vi "Calculate MF.vi"(8 "error in (no error)":errorcluster, 11 "MeritFactor in":refnum<class "MeritFactor.lvclass">) -> (0 "error out":errorcluster, 3 "MeritFactor out":refnum<class "MeritFactor.lvclass">)   [LabVIEW 2012, in "MeritFactor.lvclass"]
uses:
  MeritFactor.lvclass
  MeritFactor.lvclass/MeritFactor.ctl
  <vilib>/Analysis/baseanly.llb/Mean (DBL).vi
  <vilib>/vision/NI_Vision_Development_Module.lvlib
  <vilib>/Analysis/NI_AALBase.lvlib
panel:
  in  "Keep/Replace Value (Replace)":bool
  out "System Waveform Graph 2":T1(graph)
  out "time lapse":dbl
  out "System Waveform Graph":u32[](graph)
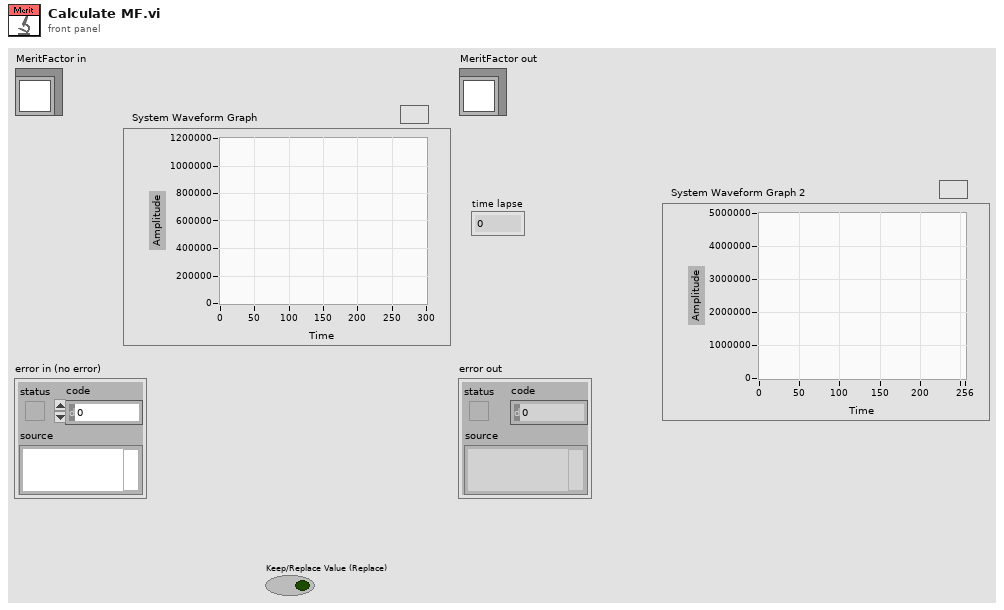
[diagram p1: front panel]
types:
  T1 = cluster{"Starting Value":sgl, "Incremental Value":sgl, "Histogram":u32[]}
  T2 = typedef "MeritFactor.lvclass/merit factor type.ctl" = enum16{"Full frame intensity", "Brightest pixels intensity", "Contrast (Keller & Stelzer)", "Contrast", "Above-threshold average"}
  T3 = typedef "IMAQ Image.ctl" = refnum<image>
  T4 = cluster{"histogram":u32[], "Minimal Value":sgl, "Maximal Value":sgl, "Starting Value":sgl, "Interval Width":sgl, "Mean Value":sgl, "Standard  Variation":sgl, "Area (pixels)":i32}
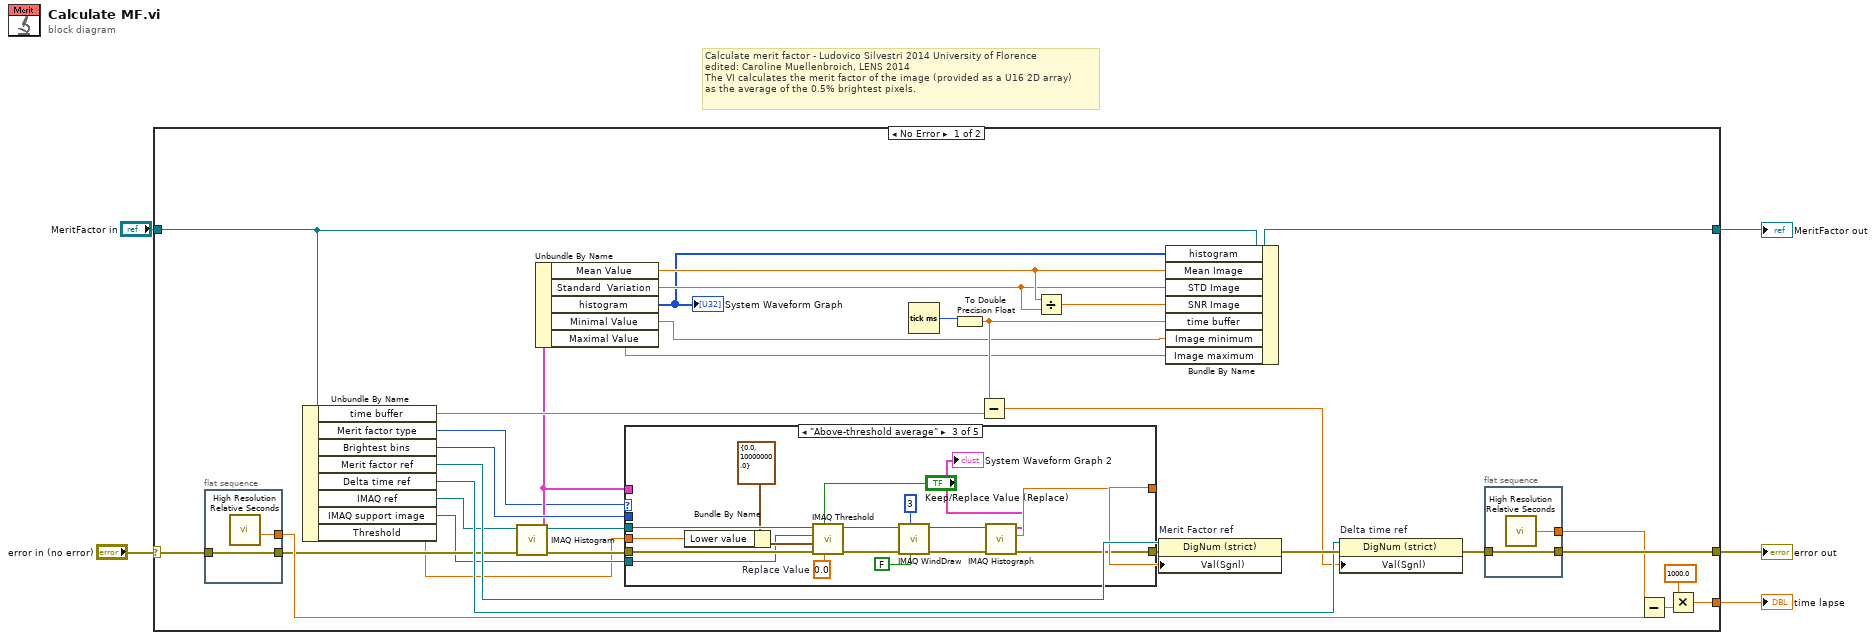
[diagram p0: block diagram]
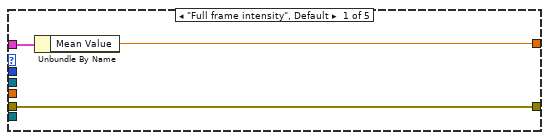
[diagram p2: hidden frame]
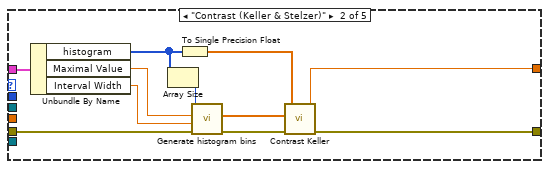
[diagram p3: hidden frame]
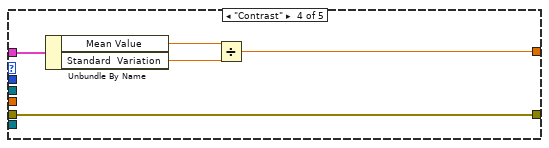
[diagram p4: hidden frame]
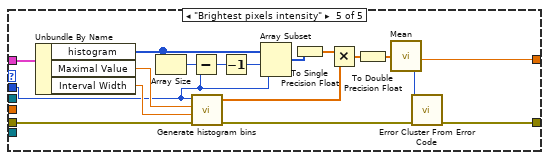
[diagram p5: hidden frame]
diagram:
  # "Calculate merit factor - Ludovico Silvestri 2014 University of Florence\nedited: Caroline Muellenbroich, LENS 2014\nThe VI calculates the merit factor of the image (provided as a U16 2D array)\nas the average of the 0.5% brightest pixels."
  n1 = case shown="No Error" "error in (no error)" {
    selector: "error in (no error)" -> [w32 w98]
    tunnel: [w30 w98] -> w4
    tunnel: [w37 w97] -> w2
    tunnel: "MeritFactor in" -> [w23 w97]
    tunnel: [w25 _] -> w1
    frame No Error {
      n2 = flat-sequence {
        tunnel: [w42] -> w28
        tunnel: w32 -> [w41]
        tunnel: [w41] -> w19
        frame #0 {
          n3 = call <vilib>:"High Resolution Relative Seconds.vi"() -> ("relative seconds"=w42:dbl)
        }
      }
      n4 = Unbundle By Name(w23) -> ("time buffer"=w18:dbl, "Merit factor type"=w11:T2, "Brightest bins"=w38:i32, "Merit factor ref"=w34:refnum<vi>, "Delta time ref"=w33:refnum<vi>, "IMAQ ref"=w8:T3, "IMAQ support image"=w7:T3, "Threshold"=w6:sgl)
      n5 = call "IMAQ Histogram"("error in (no error)"=w19, "Image"=w8) -> ("error out"=w20:errorcluster, "Histogram Report"=w14:T4)  [unwired: 8 in]
      n6 = Unbundle By Name(w14) -> ("Mean Value"=w16:sgl, "Standard  Variation"=w15:sgl, "histogram"=w12:u32[], "Minimal Value"=w10:sgl, "Maximal Value"=w9:sgl)
      "System Waveform Graph" <- w12
      n7 = case shown="\"Above-threshold average\"" w11 {
        tunnel: w20 -> [w45 w55 w73 w78 w95]
        tunnel: [w45 w47 w71 w78 w87] -> w35
        tunnel: w38 -> [_ _ _ _ w81]
        tunnel: w14 -> [w44 w56 _ w77 w96]
        tunnel: [w43 w46 w66 w74 w85] -> w13
        tunnel: w8 -> [_ _ w72 _ _]
        tunnel: w7 -> [_ _ w67 _ _]
        tunnel: w6 -> [_ _ w57 _ _]
        frame "Full frame intensity", Default {
          n8 = Unbundle By Name(w44) -> ("Mean Value"=w43:sgl)
        }
        frame "Contrast (Keller & Stelzer)" {
          n9 = Unbundle By Name(w56) -> ("histogram"=w51:u32[], "Maximal Value"=w53:sgl, "Interval Width"=w52:sgl)
          n10 = Array Size(array=w51) -> (size(s)=w54:i32)
          n11 = To Single Precision Float(number=w51) -> (single precision float=w48:sgl[])
          n12 = call "Generate histogram bins.vi"("error in (no error)"=w55, "Interval width"=w52, "Maximum value"=w53, "Brigthest bins"=w54) -> ("error out"=w50:errorcluster, "bins array"=w49:sgl[])  [unwired: 6 in]
          n13 = call "Contrast Keller.vi"("error in"=w50, "histogram bins"=w49, "histogram counts"=w48) -> ("error out"=w47:errorcluster, "Contrast"=w46:sgl)  [unwired: 7 in]
        }
        frame "Above-threshold average" {
          w70 = sgl 0.0  # Replace Value
          n14 = Bundle By Name(cluster=cluster{"Lower value":sgl, "Upper value":sgl} {"Lower value"=0.0, "Upper value"=10000000.0} ("Range"), "Lower value"=w57) -> (w68:cluster{"Lower value":sgl, "Upper value":sgl})
          n15 = call "IMAQ Threshold"("Replace Value"=w70, "Keep/Replace Value (Replace)"="Keep/Replace Value (Replace)", "error in (no error)"=w73, "Range"=w68, "Image Dst"=w67, "Image Src"=w72) -> ("error out"=w65:errorcluster, "Image Dst Out"=w62:T3)  [unwired: 4 in]
          n16 = call "IMAQ WindDraw"("Resize to Image Size? (Y)"=FALSE, "Window Number (0...15)"=3, "error in (no error)"=w65, "Image"=w62) -> ("error out"=w64:errorcluster, "Image Out (duplicate)"=w61:T3)  [unwired: 6 in]
          n17 = call "IMAQ Histograph"("error in (no error)"=w64, "Image"=w61) -> ("error out"=w71:errorcluster, "Mean Value"=w66:sgl, "Histogram Graph"=→"System Waveform Graph 2":T1)  [unwired: 6 in, 1 out]
        }
        frame "Contrast" {
          n18 = Unbundle By Name(w77) -> ("Mean Value"=w75:sgl, "Standard  Variation"=w76:sgl)
          n19 = Divide(x=w75, y=w76) -> (x/y=w74:sgl)
        }
        frame "Brightest pixels intensity" {
          n20 = Unbundle By Name(w96) -> ("histogram"=w83:u32[], "Maximal Value"=w94:sgl, "Interval Width"=w93:sgl)
          n21 = Array Size(array=w83) -> (size(s)=w82:i32)
          n22 = Subtract(x=w82, y=w81) -> (x-y=w80:i32)
          n23 = call "Generate histogram bins.vi"("error in (no error)"=w95, "Interval width"=w93, "Maximum value"=w94, "Brigthest bins"=w81) -> ("error out"=w88:errorcluster, "bins array"=w92:sgl[])  [unwired: 6 in]
          n24 = Decrement(x=w80) -> (x-1=w79:i32)
          n25 = Array Subset(array=w83, index=w79, length=w81) -> (w84:u32[])
          n26 = To Single Precision Float(number=w84) -> (single precision float=w91:sgl[])
          n27 = Multiply(x=w91, y=w92) -> (x*y=w90:sgl[])
          n28 = To Double Precision Float(number=w90) -> (double precision float=w89:dbl[])
          n29 = call-poly <vilib>:"Mean.vi"("X"=w89) -> ("mean"=w85:dbl, "error"=w86:i32)
          n30 = call <vilib>:"Error Cluster From Error Code.vi"("error in (no error)"=w88, "error code (0)"=w86) -> ("error out"=w87:errorcluster)  [unwired: 7 in]
        }
      }
      n31 = Tick Count (ms)() -> (millisecond timer value=w22:u32)
      n32 = To Double Precision Float(number=w22) -> (double precision float=w17:dbl)
      n33 = Subtract(x=w17, y=w18) -> (x-y=w21:dbl)
      n34 = Divide(x=w16, y=w15) -> (x/y=w24:sgl)
      n35 = property on="Merit Factor ref" class="DigNum (strict)"(reference=w34, error in=w35, "Val(Sgnl)"=w13) -> (error out=w36:errorcluster)  [unwired: 1 out]
      n36 = Bundle By Name(cluster=w23, "histogram"=w12, "Mean Image"=w16, "STD Image"=w15, "SNR Image"=w24, "time buffer"=w17, "Image minimum"=w10, "Image maximum"=w9) -> (w37:refnum<class "MeritFactor.lvclass">)
      n37 = property on="Delta time ref" class="DigNum (strict)"(reference=w33, error in=w36, "Val(Sgnl)"=w21) -> (error out=w31:errorcluster)  [unwired: 1 out]
      n38 = flat-sequence {
        tunnel: [w40] -> w29
        tunnel: w31 -> [w39]
        tunnel: [w39] -> w30
        frame #0 {
          n39 = call <vilib>:"High Resolution Relative Seconds.vi"() -> ("relative seconds"=w40:dbl)
        }
      }
      n40 = Subtract(x=w29, y=w28) -> (x-y=w27:dbl)
      n41 = Multiply(x=1000.0, y=w27) -> (x*y=w25:dbl)
    }
    frame Error {
    }
  }
  "error out" <- w4
  "MeritFactor out" <- w2
  "time lapse" <- w1
